vi "ClientSrv Upload.vi"(0 "file manipulation":T1, 5 "local file":path, 9 "remote file":path, 11 "error in (no error)":errorcluster, 12 "overwrite (F)":bool) -> (15 "error out":errorcluster)   [LabVIEW 2012]
doc: "Uploads a file from the client to the server. If the target file already exists it will be overwritten. To limit memory usage, the upload is performed in chunks. The duty cycle is throttled to 50% so as to not overtax the server."
uses:
  served/ClientSrv Server File Manipulation_srv.ctl
  typedefs/t_ClientSrv Server File Manipulation Methods.ctl
  typedefs/t_ClientSrv Access Levels.ctl
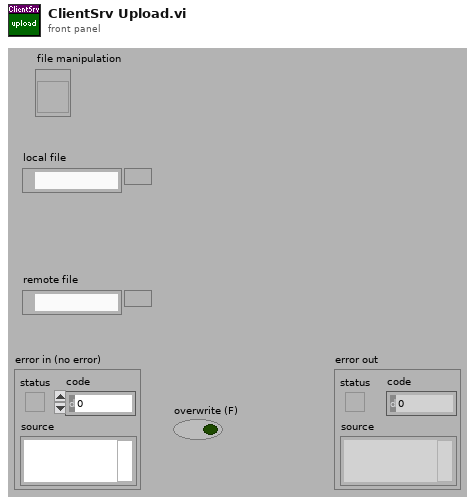
[diagram p1: front panel]
types:
  T1 = typedef "ClientSrv Server File Manipulation_srv.ctl" = refnum<vi>
  T2 = typedef "t_ClientSrv Access Levels.ctl" = enum16{"observer", "operator", "local"}
  T3 = typedef "t_ClientSrv Server File Manipulation Methods.ctl" = enum16{"close", "list", "open", "new", "read", "write", "newdir", "info", "rename", "delete"}
  T4 = enum16{"read/write", "read-only", "write-only", "write-only (truncate)"}
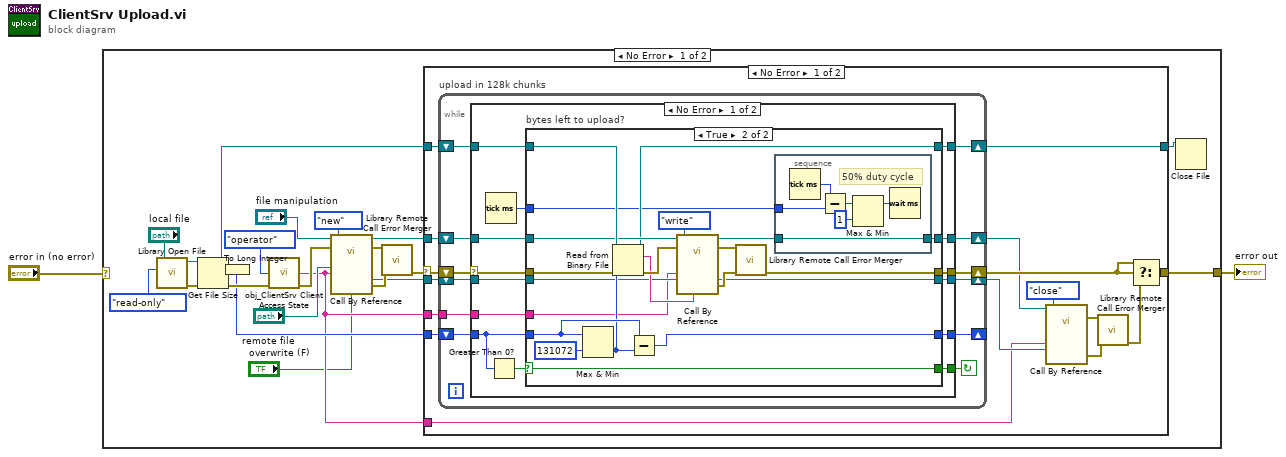
[diagram p0: block diagram]
diagram:
  n1 = case shown="No Error" "error in (no error)" {
    selector: "error in (no error)" -> [_ w107]
    tunnel: [w6 w107] -> w2
    frame No Error {
      n2 = call "Library Open File.vi"("open mode (read/write)"=T4."read-only", "file path"="local file") -> ("error out"=w22:errorcluster, "refnum"=w21:refnum<file>)  [unwired: 4 in]
      n3 = Get File Size(file=w21, error in=w22) -> (refnum out=w10:refnum<file>, size (in bytes)=w3:i64, 0:w20:errorcluster)
      n4 = To Long Integer(number=w3) -> (32bit integer=w11:i32)
      n5 = call "obj_ClientSrv Client Access State.vi"("access level (observer)"=t_ClientSrv_Access_Levels."operator", "error in (no error)"=w20) -> ("certificate"=w5:string, "error out"=w18:errorcluster)  [unwired: 12 in]
      n6 = call-by-ref "?"(reference="file manipulation", error in=w18, "method"=t_ClientSrv_Server_File_Manipulation_Methods."new", "path"="remote file", "certificate"=w5, "overwrite (F)"="overwrite (F)") -> (reference out=w8:T1, error out=w15:errorcluster, "refnum out"=w12:refnum<file>, 15:"error out"=w14:errorcluster)  [unwired: 4 in, 6 out]
      n7 = call "Library Remote Call Error Merger.vi"("call by reference node error"=w15, "called VI error (no error)"=w14) -> ("error out"=w13:errorcluster)  [unwired: 13 in]
      n8 = case shown="No Error" w13 {
        selector: w13 -> [w35 w105]
        tunnel: w12 -> [w36 _]
        tunnel: w11 -> [w39 _]
        tunnel: w10 -> [w40 w106]
        tunnel: [w38 w106] -> w9
        tunnel: w8 -> [w37 _]
        tunnel: [w28 w105] -> w6
        tunnel: w5 -> [w26 _]
        tunnel: w5 -> [w25 _]
        frame No Error {
          n9 = while "upload in 128k chunks" {
            shift-right: [w48] -> w38
            shift-left: w40 -> [w49]
            shift-right: [w46] -> _
            shift-left: w39 -> [w52]
            shift-right: [w44] -> w27
            shift-left: w37 -> [w45]
            shift-right: [w42] -> w33
            shift-left: w36 -> [w43]
            shift-right: [w50] -> w30
            shift-left: w35 -> [w51]
            tunnel: w26 -> [w41]
            stop <- w47 continue-if-true
            n10 = case shown="No Error" w51 {
              selector: w51 -> [w60 w104]
              tunnel: w52 -> [w63 w102]
              tunnel: [w56 w104] -> w50
              tunnel: [w57 w103] -> w48
              tunnel: w49 -> [w61 w103]
              tunnel: [w65 _] -> w47
              tunnel: w41 -> [w64 _]
              tunnel: [w62 w102] -> w46
              tunnel: w45 -> [w59 w101]
              tunnel: [w58 w101] -> w44
              tunnel: w43 -> [w54 w100]
              tunnel: [w53 w100] -> w42
              frame No Error {
                n11 = Tick Count (ms)() -> (millisecond timer value=w55:u32)
                n12 = Greater Than 0?(x=w63) -> (x > 0?=w66:bool)
                n13 = case "bytes left to upload?" shown="True" w66 {
                  selector: w66 -> [w72 w93]
                  tunnel: [w72 w93] -> w65
                  tunnel: w64 -> [_ w73]
                  tunnel: w63 -> [w71 w89]
                  tunnel: [w71 w88] -> w62
                  tunnel: w61 -> [w69 w92]
                  tunnel: w60 -> [w68 w91]
                  tunnel: w59 -> [w70 w86]
                  tunnel: [w70 w78] -> w58
                  tunnel: [w69 w77] -> w57
                  tunnel: [w68 w80] -> w56
                  tunnel: w55 -> [_ w76]
                  tunnel: w54 -> [w67 w75]
                  tunnel: [w67 w74] -> w53
                  frame False {
                  }
                  frame True {
                    n14 = Max & Min(x=w89, y=131072) -> (min(x,y)=w87:i32)  [unwired: 1 out]
                    n15 = Read from Binary File(8:w91, 10:w87, 11:w92) -> (0:w84:errorcluster, 2:w81:string, 3:w77:refnum<file>)  [unwired: 3 in, 1 out]
                    n16 = Subtract(x=w89, y=w87) -> (x-y=w88:i32)
                    n17 = call-by-ref "?"(reference=w86, error in=w84, "method"=t_ClientSrv_Server_File_Manipulation_Methods."write", "certificate"=w73, "refnum in"=w75, "data in"=w81) -> (reference out=w79:T1, error out=w83:errorcluster, "refnum out"=w74:refnum<file>, 15:"error out"=w82:errorcluster)  [unwired: 4 in, 6 out]
                    n18 = call "Library Remote Call Error Merger.vi"("call by reference node error"=w83, "called VI error (no error)"=w82) -> ("error out"=w80:errorcluster)  [unwired: 13 in]
                    n19 = stacked-sequence {
                      tunnel: w79 -> [w99]
                      tunnel: [w99] -> w78
                      tunnel: w76 -> [w98]
                      frame #0 {
                        # "50% duty cycle"
                        n20 = Tick Count (ms)() -> (millisecond timer value=w97:u32)
                        n21 = Subtract(x=w97, y=w98) -> (x-y=w96:u32)
                        n22 = Max & Min(x=w96, y=u32 1) -> (max(x,y)=w94:u32)  [unwired: 1 out]
                        n23 = Wait (ms)(milliseconds to wait=w94) -> ()  [unwired: 1 out]
                      }
                    }
                  }
                }
              }
              frame Error {
              }
            }
          }
          n24 = call-by-ref "?"(reference=w27, "method"=t_ClientSrv_Server_File_Manipulation_Methods."close", "certificate"=w25, "refnum in"=w33) -> (error out=w32:errorcluster, 15:"error out"=w31:errorcluster)  [unwired: 6 in, 8 out]
          n25 = call "Library Remote Call Error Merger.vi"("call by reference node error"=w32, "called VI error (no error)"=w31) -> ("error out"=w29:errorcluster)  [unwired: 13 in]
          n26 = Select(t=w30, s=w30, f=w29) -> (s? t:f=w28:errorcluster)
        }
        frame Error {
        }
      }
      n27 = Close File(refnum=w9) -> ()  [unwired: 1 in, 2 out]
    }
    frame Error {
    }
  }
  "error out" <- w2
